vi "ReadSampleNode.vi"(8 "Error In":errorcluster, 11 "Experiment Node In":refnum<k20>) -> (0 "Error Out":errorcluster, 2 "Sample":T1, 3 "Experiment Node Out":refnum<k20>)   [LabVIEW 2012]
uses:
  Sample.ctl
  <vilib>/xml/NI_XML.lvlib
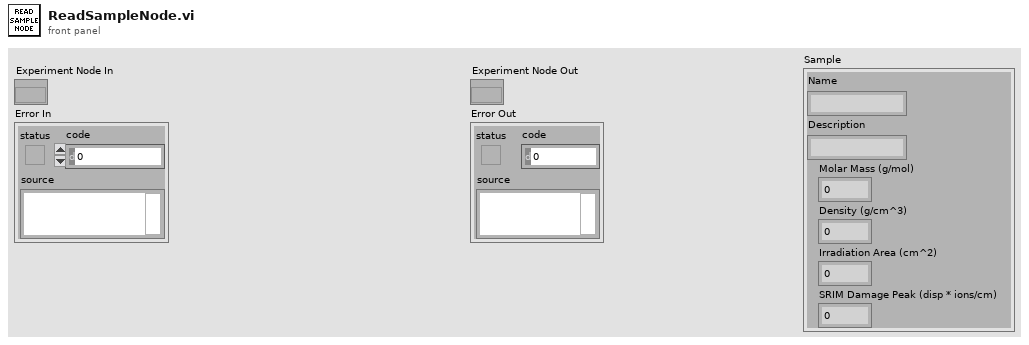
[diagram p1: front panel]
types:
  T1 = typedef "Sample.ctl" = cluster{"Name":string, "Description":string, "Molar Mass (g/mol)":dbl, "Density (g/cm^3)":dbl, "Irradiation Area (cm^2)":dbl, "SRIM Damage Peak (disp * ions/cm)":dbl}
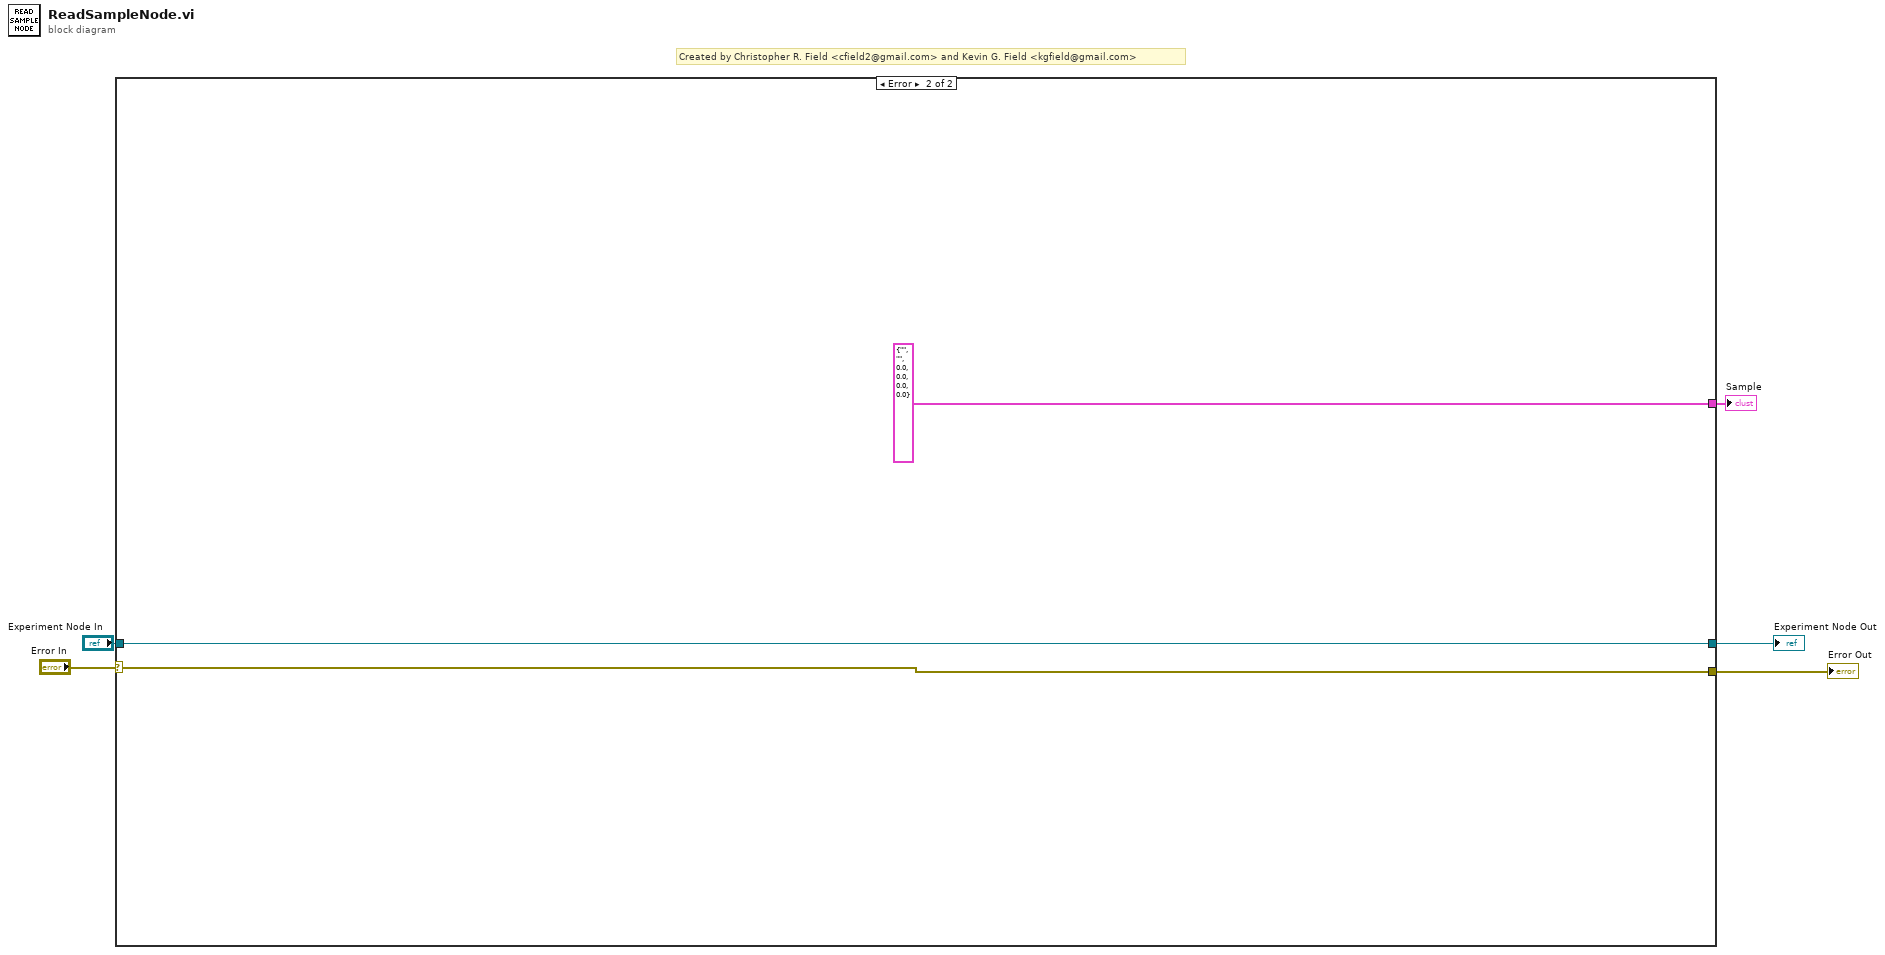
[diagram p0: block diagram]
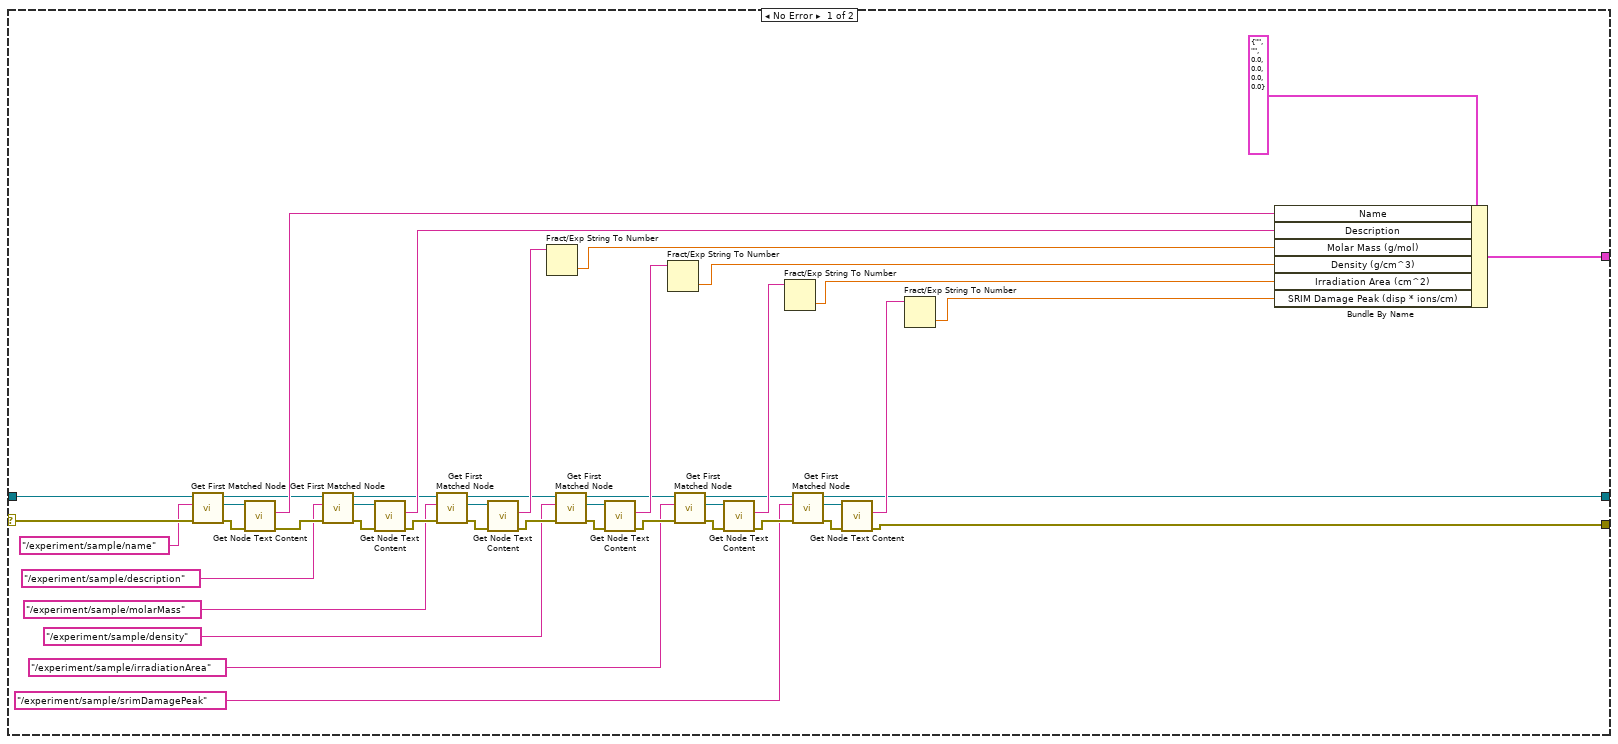
[diagram p2: hidden frame]
diagram:
  # "Created by Christopher R. Field <cfield2@gmail.com> and Kevin G. Field <kgfield@gmail.com>"
  n1 = case shown="Error" "Error In" {
    selector: "Error In" -> [w48 w51]
    tunnel: "Experiment Node In" -> [w49 w52]
    tunnel: [w7 w52] -> w3
    tunnel: [w6 w51] -> w2
    tunnel: [w43 T1 {"Name"="", "Description"="", "Molar Mass (g/mol)"=0.0, "Density (g/cm^3)"=0.0, "Irradiation Area (cm^2)"=0.0, "SRIM Damage Peak (disp * ions/cm)"=0.0} ("Sample")] -> w1
    frame No Error {
      n2 = call <vilib>:"Get First Matched Node.vi"("error in (no error)"=w48, "XPath expression"="/experiment/sample/name", "node in"=w49) -> ("error out"=w45:errorcluster, "node result"=w46:refnum<k20>, "node out"=w41:refnum<k20>)  [unwired: 6 in]
      n3 = call <vilib>:"Get Node Text Content.vi"("error in (no error)"=w45, "node in"=w46) -> ("error out"=w40:errorcluster, "node text"=w42:string)  [unwired: 7 in, 1 out]
      n4 = call <vilib>:"Get First Matched Node.vi"("error in (no error)"=w40, "XPath expression"="/experiment/sample/description", "node in"=w41) -> ("error out"=w37:errorcluster, "node result"=w38:refnum<k20>, "node out"=w35:refnum<k20>)  [unwired: 6 in]
      n5 = call <vilib>:"Get Node Text Content.vi"("error in (no error)"=w37, "node in"=w38) -> ("error out"=w34:errorcluster, "node text"=w36:string)  [unwired: 7 in, 1 out]
      n6 = call <vilib>:"Get First Matched Node.vi"("error in (no error)"=w34, "XPath expression"="/experiment/sample/molarMass", "node in"=w35) -> ("error out"=w31:errorcluster, "node result"=w32:refnum<k20>, "node out"=w28:refnum<k20>)  [unwired: 6 in]
      n7 = call <vilib>:"Get Node Text Content.vi"("error in (no error)"=w31, "node in"=w32) -> ("error out"=w27:errorcluster, "node text"=w30:string)  [unwired: 7 in, 1 out]
      n8 = Fract/Exp String To Number(string=w30) -> (number=w29:dbl)  [unwired: 3 in, 1 out]
      n9 = call <vilib>:"Get First Matched Node.vi"("error in (no error)"=w27, "XPath expression"="/experiment/sample/density", "node in"=w28) -> ("error out"=w24:errorcluster, "node result"=w25:refnum<k20>, "node out"=w19:refnum<k20>)  [unwired: 6 in]
      n10 = call <vilib>:"Get Node Text Content.vi"("error in (no error)"=w24, "node in"=w25) -> ("error out"=w18:errorcluster, "node text"=w23:string)  [unwired: 7 in, 1 out]
      n11 = Fract/Exp String To Number(string=w23) -> (number=w22:dbl)  [unwired: 3 in, 1 out]
      n12 = call <vilib>:"Get First Matched Node.vi"("error in (no error)"=w18, "XPath expression"="/experiment/sample/irradiationArea", "node in"=w19) -> ("error out"=w20:errorcluster, "node result"=w21:refnum<k20>, "node out"=w12:refnum<k20>)  [unwired: 6 in]
      n13 = call <vilib>:"Get Node Text Content.vi"("error in (no error)"=w20, "node in"=w21) -> ("error out"=w11:errorcluster, "node text"=w16:string)  [unwired: 7 in, 1 out]
      n14 = Fract/Exp String To Number(string=w16) -> (number=w15:dbl)  [unwired: 3 in, 1 out]
      n15 = call <vilib>:"Get First Matched Node.vi"("error in (no error)"=w11, "XPath expression"="/experiment/sample/srimDamagePeak", "node in"=w12) -> ("error out"=w13:errorcluster, "node result"=w14:refnum<k20>, "node out"=w7:refnum<k20>)  [unwired: 6 in]
      n16 = call <vilib>:"Get Node Text Content.vi"("error in (no error)"=w13, "node in"=w14) -> ("error out"=w6:errorcluster, "node text"=w9:string)  [unwired: 7 in, 1 out]
      n17 = Fract/Exp String To Number(string=w9) -> (number=w8:dbl)  [unwired: 3 in, 1 out]
      n18 = Bundle By Name(cluster=T1 {"Name"="", "Description"="", "Molar Mass (g/mol)"=0.0, "Density (g/cm^3)"=0.0, "Irradiation Area (cm^2)"=0.0, "SRIM Damage Peak (disp * ions/cm)"=0.0} ("Sample"), "Name"=w42, "Description"=w36, "Molar Mass (g/mol)"=w29, "Density (g/cm^3)"=w22, "Irradiation Area (cm^2)"=w15, "SRIM Damage Peak (disp * ions/cm)"=w8) -> (w43:T1)
    }
    frame Error {
    }
  }
  "Experiment Node Out" <- w3
  "Error Out" <- w2
  "Sample" <- w1
